vi "visionCalcs.vi"(10 "Vision Angle?":bool, 11 "Vision Distance?":bool) -> (3 "angle":dbl)   [LabVIEW 2017, in "Apple script.lvlib"]
uses:
  AppleScript/Apple script.lvlib
  <vilib>/Rock Robotics/Network Tables/NT Read Number.vi
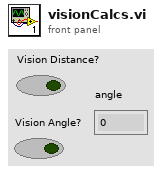
[diagram p1: front panel]
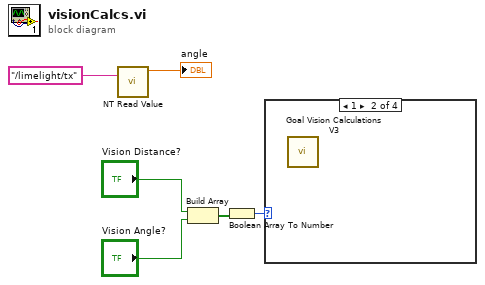
[diagram p0: block diagram]
diagram:
  n1 = call-poly <vilib>:"NT Read Value.vi"("Name"="/limelight/tx") -> ("Numeric"=→"angle":dbl)  [unwired: 9 in, 1 out]
  n2 = Build Array("Vision Distance?", "Vision Angle?") -> (w4:bool[])
  n3 = Boolean Array To Number(Boolean array=w4) -> (number=w3:u32)
  n4 = case shown="1" w3 {
    frame 0, Default {
    }
    frame 1 {
      n5 = call "Goal Vision Calculations V3.vi"() -> ()  [unwired: 9 in, 2 out]
    }
    frame 2 {
    }
    frame 3 {
    }
  }
